vi "home.vi"(8 "error in (no error)":errorcluster, 11 "imaginaryStage in":refnum<class "imaginaryStage.lvclass">) -> (0 "error out":errorcluster, 3 "imaginaryStage out":refnum<class "imaginaryStage.lvclass">)   [LabVIEW 2019, in "imaginaryStage.lvclass"]
uses:
  imaginaryStage.lvclass
  _delayStageBase/_delayStageBase.lvclass
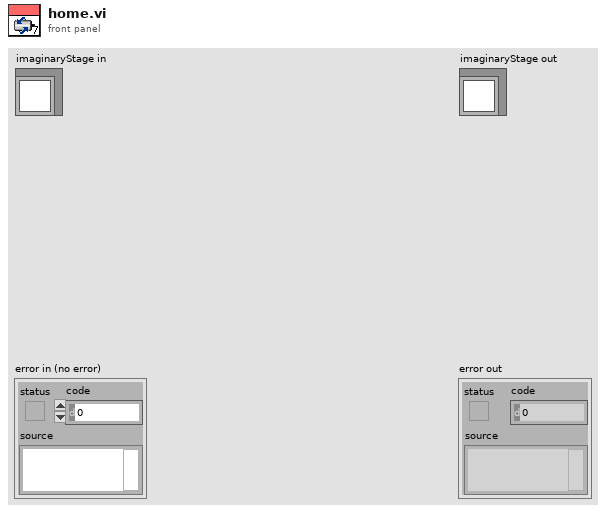
[diagram p1: front panel]
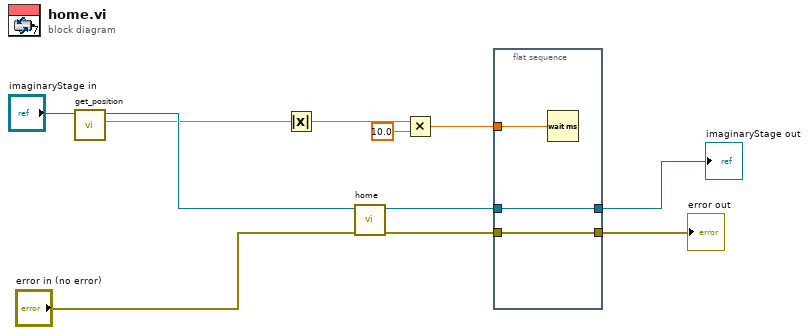
[diagram p0: block diagram]
diagram:
  n1 = call-dynamic "get_position.vi"("_delayStageBase in"="imaginaryStage in") -> ("last position"=w8:dbl, "_delayStageBase out"=w9:refnum<class "imaginaryStage.lvclass">)  [unwired: 8 in, 1 out]
  n2 = Absolute Value(x=w8) -> (abs(x)=w3:dbl)
  n3 = call-parent "home.vi"("error in (no error)"="error in (no error)", "_delayStageBase in"=w9) -> ("error out"=w4:errorcluster, "_delayStageBase out"=w7:refnum<class "imaginaryStage.lvclass">)  [unwired: 8 in]
  n4 = Multiply(x=w3, y=10.0) -> (x*y=w1:dbl)
  n5 = flat-sequence {
    tunnel: w7 -> [w14]
    tunnel: [w14] -> w6
    tunnel: [w13] -> w5
    tunnel: w4 -> [w13]
    tunnel: w1 -> [w12]
    frame #0 {
      n6 = Wait (ms)(milliseconds to wait=w12) -> ()  [unwired: 1 out]
    }
  }
  "error out" <- w5
  "imaginaryStage out" <- w6
